vi "Convert Frame to NI-XNET CAN Frame.vi"(8 "error in (no error)":errorcluster, 11 "Data to Send":T1 {"Identifier" format="%08x"}) -> (0 "error out":errorcluster, 3 "CAN frame":T2 {"payload" format="%x"; "timestamp" format="%<%.7X\n%x>T"; "type" items=["CAN Data"=0, "CAN Remote"=1, "CAN Bus Error"=2, "Delay"=224, "Log Trigger"=225, "Start Trigger"=226]; "identifier" format="%x"})   [LabVIEW 2013, in "J1939 Addon Engine.lvlib"]
uses:
  Engine/J1939 Addon Engine.lvlib
  <vilib>/xnet/xnet.llb/XNET Frame CAN.ctl
  <vilib>/xnet/xnet.llb/XNET Frame Type CAN.ctl
  J1939 Utilities/Types/CAN Outgoing Message Cluster.ctl
  J1939 Utilities/J1939 Utilities.lvlib
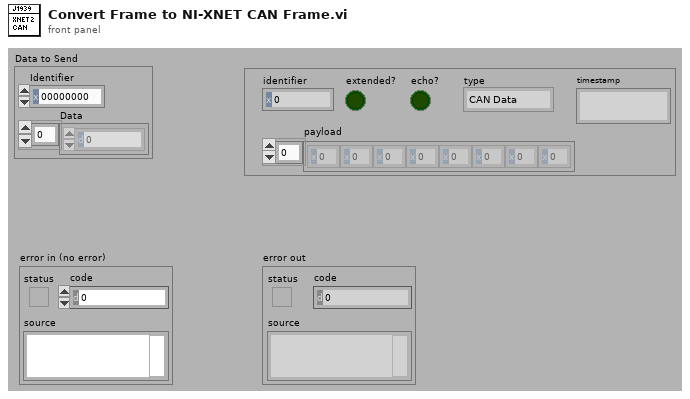
[diagram p1: front panel]
types:
  T1 = typedef "J1939 Addon Shared.lvlib/J1939 Utilities.lvlib/CAN Outgoing Message Cluster.ctl" = cluster{"Identifier":u32, "Data":u8[]}
  T2 = typedef "XNET Frame CAN.ctl" = cluster{"timestamp":timestamp, "payload":u8[], "identifier":u32, "type":T3, "extended?":bool, "echo?":bool}
  T3 = typedef "XNET Frame Type CAN.ctl" = u8
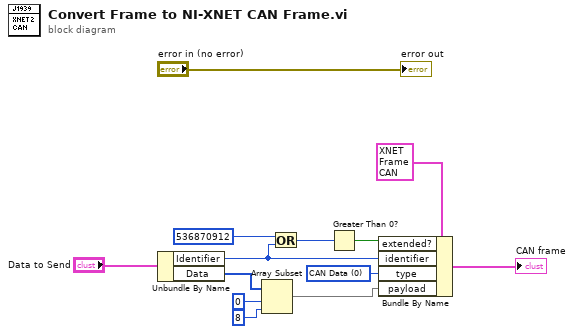
[diagram p0: block diagram]
diagram:
  w2 = T3 0 items=["CAN Data", "CAN Remote"] ("type")
  n1 = Unbundle By Name("Data to Send") -> ("Identifier"=w9:u32, "Data"=w5:u8[])
  n2 = Array Subset(array=w5, index=0, length=8) -> (w4:u8[])
  n3 = Or(x=u32 536870912, y=w9) -> (x .or. y?=w11:u32)
  n4 = Greater Than 0?(x=w11) -> (x > 0?=w8:bool)
  n5 = Bundle By Name(cluster=T2 {"timestamp"=timestamp(0 s since 1904-01-01), "payload"=[], "identifier"=0, "type"=0, "extended?"=FALSE, "echo?"=FALSE} ("CAN frame"), "extended?"=w8, "identifier"=w9, "type"=w2, "payload"=w4) -> (→"CAN frame":T2)
  "error out" <- "error in (no error)"
